vi "Log and Create New if Required.vi"(0 "event data in":T2, 5 "log data":T1[](array[typedef]), 11 "error in":errorcluster) -> (4 "event data out":T2, 15 "error out":errorcluster)   [LabVIEW 2021, in "Event Logger.lvlib"]
uses:
  Event Logger.lvlib
  TypeDefs/Event Data Cluster.ctl
  TypeDefs/Event Values.ctl
  <vilib>/Utility/file.llb/Write Delimited Spreadsheet (string).vi
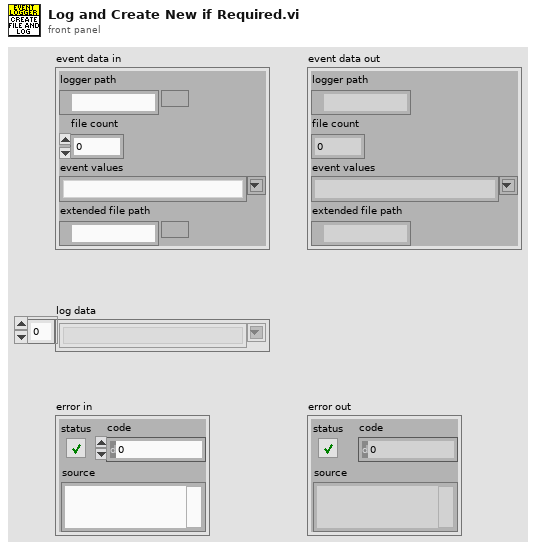
[diagram p1: front panel]
types:
  T1 = typedef "Event Logger.lvlib/Event Values.ctl" = string
  T2 = typedef "Event Logger.lvlib/Event Data Cluster.ctl" = cluster{"logger path":path, "file count":i32, "event values":T1, "extended file path":path}
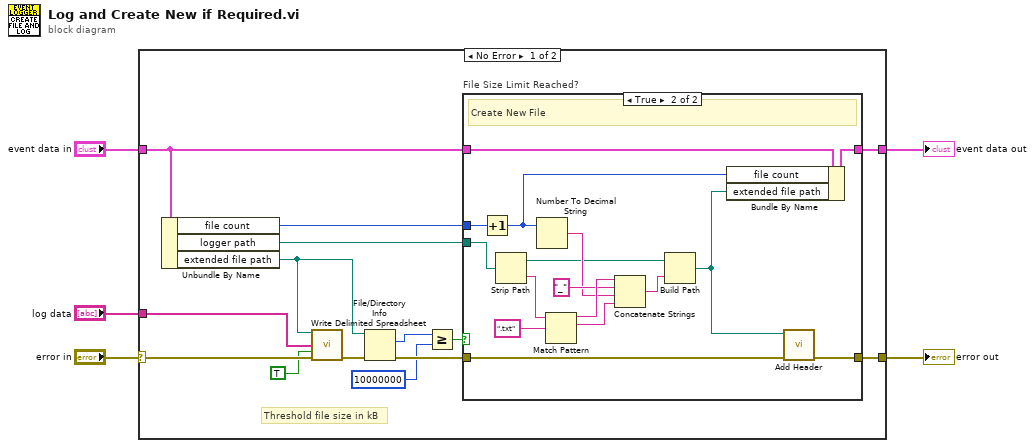
[diagram p0: block diagram]
diagram:
  n1 = case shown="No Error" "error in" {
    selector: "error in" -> [w12 w39]
    tunnel: [w19 w38] -> w5
    tunnel: [w18 w39] -> w4
    tunnel: "event data in" -> [w14 w38]
    tunnel: "log data" -> [w10 _]
    frame No Error {
      # "Threshold file size in kB"
      n2 = Unbundle By Name(w14) -> ("file count"=w13:i32, "logger path"=w8:path, "extended file path"=w7:path)
      n3 = call-poly <vilib>:"Write Delimited Spreadsheet.vi"("file path (dialog if empty)"=w7, "1D data"=w10, "append to file? (new file:F)"=TRUE, "error in (no error)"=w12) -> ("error out"=w11:errorcluster)  [unwired: 10 in, 1 out]
      n4 = File/Directory Info(path=w7, error in=w11) -> (size=w15:i64, error out=w16:errorcluster)  [unwired: 5 out]
      n5 = Greater Or Equal?(x=w15, y=i64 10000000) -> (x >= y?=w17:bool)
      n6 = case "File Size Limit Reached?" shown="True" w17 {
        tunnel: w16 -> [w21 w24]
        tunnel: [w21 w25] -> w18
        tunnel: w13 -> [_ w35]
        tunnel: w14 -> [w20 w29]
        tunnel: [w20 w28] -> w19
        tunnel: w8 -> [_ w23]
        frame False {
          # "Use the same file"
        }
        frame True {
          # "Create New File"
          n7 = Increment(x=w35) -> (x+1=w27:i32)
          n8 = Strip Path(path=w23) -> (stripped path=w31:path, name=w37:string)
          n9 = Number To Decimal String(number=w27) -> (decimal integer string=w32:string)  [unwired: 1 in]
          n10 = Match Pattern(string=w37, regular expression=".txt") -> (before substring=w34:string, match substring=w22:string)  [unwired: 1 in, 2 out]
          n11 = Concatenate Strings(w34, "_" ("string"), w32, w22) -> (w30:string)
          n12 = Build Path(base path=w31, name or relative path=w30) -> (appended path=w26:path)
          n13 = Bundle By Name(cluster=w29, "file count"=w27, "extended file path"=w26) -> (w28:T2)
          n14 = call "Add Header.vi"("error in"=w24, "logger path"=w26) -> ("error out"=w25:errorcluster)  [unwired: 9 in]
        }
      }
    }
    frame Error {
    }
  }
  "event data out" <- w5
  "error out" <- w4
